vi "lift setpoint driver control.vi"(1 "Current Setpoint":dbl, 3 "Joystick Y":dbl) -> (0 "Setpoint":dbl)   [LabVIEW 2014]
uses:
  global variables/devrefs.vi
panel:
  # "Control the lift with PID setpoints instead of direct motor control"
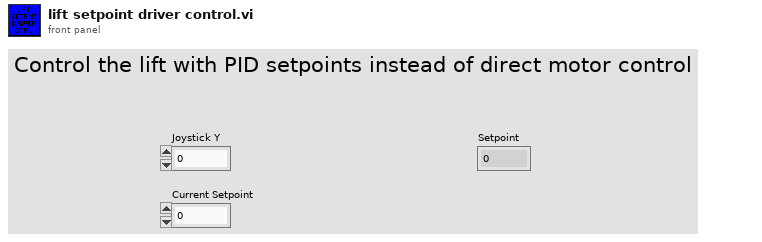
[diagram p1: front panel]
types:
  T1 = typedef "WPI_EncoderDevRef.ctl" = cluster{"DevStatus":errorcluster, "EncoderIndex":T2, "CounterIndex":T3, "DistancePerCount":dbl, "Decoding Type":T4}
  T2 = typedef "FPGA_EncoderIdx.ctl" = enum8{"Enc 0", "Enc 1", "Enc 2", "Enc 3", "Enc 4", "Enc 5", "Enc 6", "Enc 7", "Invalid"}
  T3 = typedef "FPGA_CounterCtrSystemIndex.ctl" = enum8{"Ctr 0", "Ctr 1", "Ctr 2", "Ctr 3", "Ctr 4", "Ctr 5", "Ctr 6", "Ctr 7", "Invalid"}
  T4 = typedef "WPI_EncoderType.ctl" = enum16{"1x", "2x", "4x"}
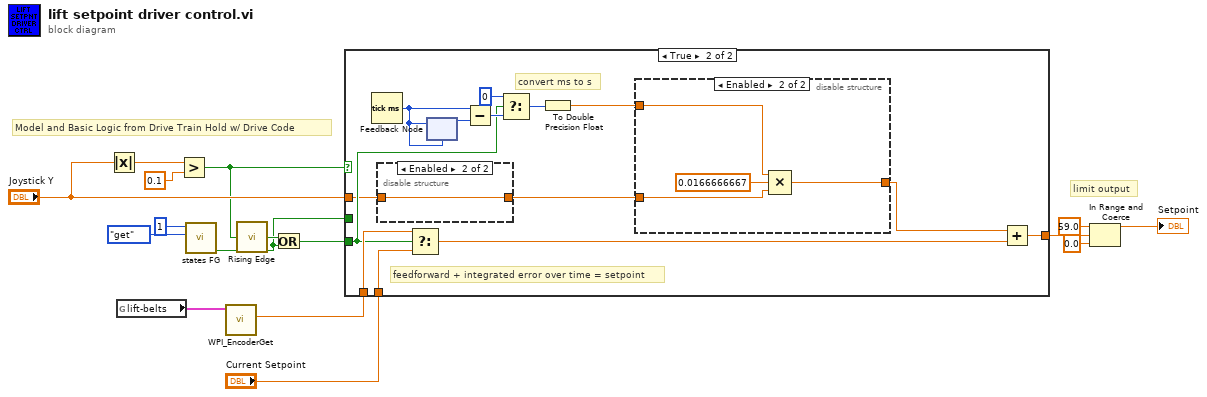
[diagram p0: block diagram]
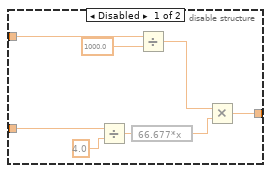
[diagram p4: hidden frame]
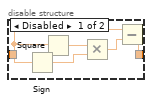
[diagram p5: hidden frame]
diagram:
  # "limit output"
  # "Model and Basic Logic from Drive Train Hold w/ Drive Code"
  n1 = Absolute Value(x="Joystick Y") -> (abs(x)=w16:dbl)
  n2 = global read "devrefs.vi" "lift-belts"() -> (w6:T1)
  n3 = Greater?(x=w16, y=0.1) -> (0:w10:bool)
  n4 = call "states FG.vi"("menu (get)"=enum16{"set", "get"}."get", "Loop ID"=1) -> ("first call?"=w7:bool)  [unwired: 6 in, 3 out]
  n5 = call <vilib>:"WPI_EncoderGet.vi"("EncoderDevRef"=w6) -> ("Distance"=w9:dbl)  [unwired: 5 in, 5 out]
  n6 = call "Rising Edge.vi"("Input"=w10) -> ("Rising Edge"=w12:bool)
  n7 = Or(x=w12, y=w7) -> (x .or. y?=w8:bool)
  n8 = case shown="True" w10 {
    tunnel: "Joystick Y" -> [_ w29]
    tunnel: "Current Setpoint" -> [w20 w34]
    tunnel: w8 -> [_ w30]
    tunnel: w9 -> [w19 w33]
    tunnel: [w18 w27] -> w3
    tunnel: w7 -> [w17 _]
    frame False {
      n9 = case shown="False" w17 {
        tunnel: w20 -> [w21 _]
        tunnel: w19 -> [_ w22]
        tunnel: [w21 w22] -> w18
        frame False {
          # "and get it there if it isn't there"
          # "hold lift at current commanded location"
        }
        frame True {
          # "hold lift at encoder location"
        }
      }
    }
    frame True {
      # "feedforward + integrated error over time = setpoint"
      # "convert ms to s"
      n10 = Tick Count (ms)() -> (millisecond timer value=w24:u32)
      n11 = disable-structure shown="Enabled" {
        disable-tunnel: w29 -> [w53 w54]
        disable-tunnel: [w52 w54] -> w26
        frame Disabled {
          n12 = Sign(1:w53) -> (0:w50:dbl)
          n13 = Square(x=w53) -> (x^2=w51:dbl)
          n14 = Multiply(x=w51, y=w50) -> (x*y=w49:dbl)
          n15 = Subtract(x=w53, y=w49) -> (x-y=w52:dbl)
        }
        frame Enabled {
        }
      }
      n16 = Select(t=w33, s=w30, f=w34) -> (s? t:f=w28:dbl)
      n17 = feedback #1(w24) -> (w25:u32)
      n18 = feedback-in #1(w24) -> ()
      n19 = Subtract(x=w24, y=w25) -> (x-y=w35:u32)
      n20 = Select(t=u32 0, s=w30, f=w35) -> (s? t:f=w31:u32)
      n21 = To Double Precision Float(number=w31) -> (double precision float=w32:dbl)
      n22 = disable-structure shown="Enabled" {
        disable-tunnel: w32 -> [w44 w48]
        disable-tunnel: w26 -> [w40 w47]
        disable-tunnel: [w37 w45] -> w23
        frame Disabled {
          n23 = Divide(x=w40, y=4.0) -> (x/y=w39:dbl)
          n24 = expression code="66.677*x"(w39) -> (w38:dbl)
          n25 = Divide(x=w44, y=1000.0) -> (x/y=w42:dbl)
          n26 = Multiply(x=w42, y=w38) -> (x*y=w37:dbl)
        }
        frame Enabled {
          n27 = Compound Arithmetic op=MULTIPLY(w48, 0.0166666667 ("value"), w47) -> (w45:dbl)
        }
      }
      n28 = Add(x=w23, y=w28) -> (x+y=w27:dbl)
    }
  }
  n29 = In Range and Coerce(upper limit=59.0, x=w3, lower limit=0.0) -> (coerced(x)=→"Setpoint":dbl)  [unwired: 1 out]
